vi "UIRef.vi"(8 "error in":errorcluster, 11 "PC in":refnum<class "PLTarget PC.lvclass">) -> (0 "error out":errorcluster, 2 "VI refnum":refnum<vi>, 3 "PC out":refnum<class "PLTarget PC.lvclass">)   [LabVIEW 2013, in "PLTarget PC.lvclass"]
doc: "Stores the static reference to the UI of the node."
uses:
  PLTarget PC.lvclass
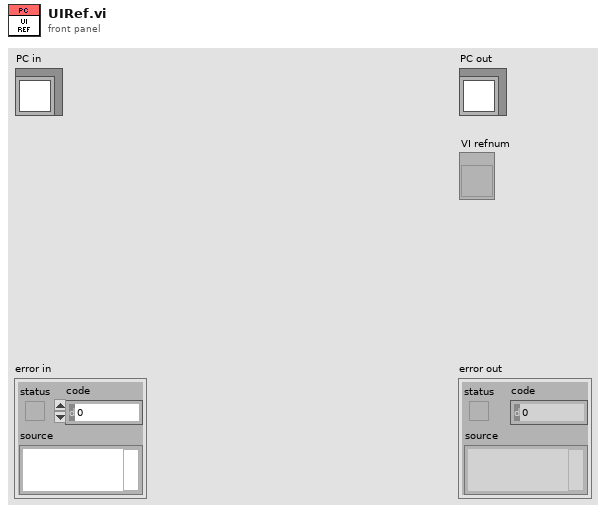
[diagram p1: front panel]
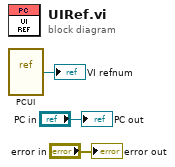
[diagram p0: block diagram]
diagram:
  n1 = vi-ref "PCUI.vi"() -> (→"VI refnum":refnum<vi>)
  "error out" <- "error in"
  "PC out" <- "PC in"
